vi "Connect Channel Command.vi"(8 "error in":errorcluster, 10 "Channel Connection Data":T1 {"Connection Data" format="%x"}, 11 "CIFCorePlugin in":refnum<class "CIFCorePlugin.lvclass">) -> (0 "error out":errorcluster, 3 "CIFCorePlugin out":refnum<class "CIFCorePlugin.lvclass">)   [LabVIEW 2021, in "CIFCorePlugin.lvclass"]
uses:
  CIFCorePlugin.lvclass
  CIFCorePlugin.lvclass/CIFCorePlugin.ctl
  Typedef/gRPC to Main Commands.ctl
  7fb4bced-bf7d-48d6-a5d3-7671888d20d0.vi
  Typedef/gRPC to Main Command Payload.ctl
  Common/Typedef/Channel Connection Data.ctl
  Common/CIFCoreCommon.lvlib
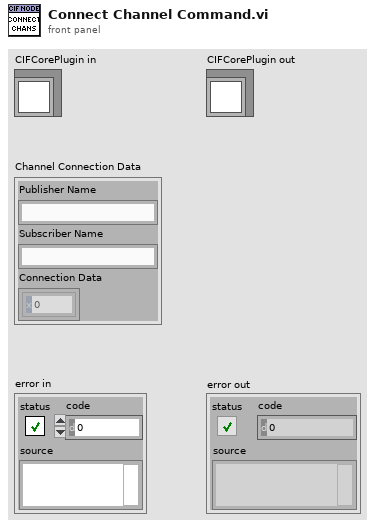
[diagram p1: front panel]
types:
  T1 = typedef "CIFCoreCommon.lvlib/Channel Connection Data.ctl" = cluster{"Publisher Name":string, "Subscriber Name":string, "Connection Data":u8[]}
  T2 = typedef "gRPC to Main Command Payload.ctl" = cluster{"OOB_Rx Command":T3, "Array Index":i32}
  T3 = typedef "CIFCorePlugin.lvclass/gRPC to Main Commands.ctl" = enum8{"Start", "Pause", "Stop", "RefreshStats", "UpdateConfig", "Update Clock Map", "Connect Channel", "Force Channel", "Add Publisher Instance", "Remove Publisher Instance"}
  T4 = typedef "CIFCorePlugin.lvclass/gRPC to Main DVR.ctl" = refnum<data-value>
  T5 = typedef "CIFCoreCommon.lvlib/gRPC to Main Data.ctl" = cluster{"Config Data":variant, "Connections":T1[], "Forces":T6[], "Clock Conversion":T7, "Publisher Instance":T9}
  T6 = typedef "CIFCoreCommon.lvlib/Channel Force Data.ctl" = cluster{"Channel Name":string, "Force Data":u8[], "Force Active":bool}
  T7 = typedef "Time_CIF_U.lvlib/Clock Conversion Map.ctl" = map{u8, cluster{"Last Reset":i64, "Offset Pair":T8, "Slope":dbl, "1/Slope":dbl}}
  T8 = typedef "Time_CIF_U.lvlib/Timestamp Pair.ctl" = cluster{"System Time":i64, "External Time":i64}
  T9 = typedef "CIFCoreCommon.lvlib/FIFO Publisher.ctl" = cluster{"Publisher Name":string, "New FIFO Instance Config":T10}
  T10 = typedef "ChannelCommon.lvlib/New FIFO Instance Configuration.ctl" = cluster{"Primary":bool, "Backpressure":bool, "Message/FIFO Override":u32}
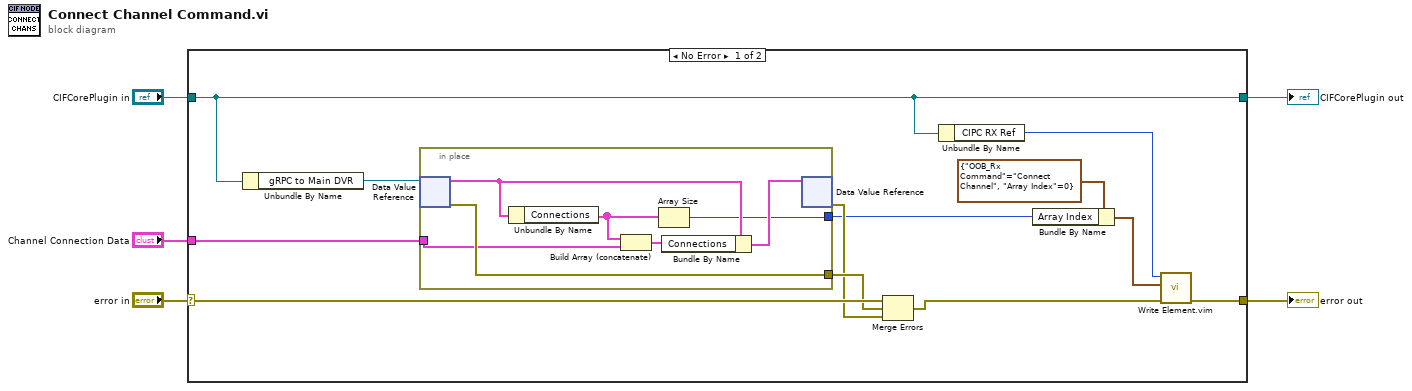
[diagram p0: block diagram]
diagram:
  n1 = case shown="No Error" "error in" {
    selector: "error in" -> [w12 w26]
    tunnel: [w17 w26] -> w4
    tunnel: "CIFCorePlugin in" -> [w15 w25]
    tunnel: [w15 w25] -> w2
    tunnel: "Channel Connection Data" -> [w13 _]
    frame No Error {
      n2 = Unbundle By Name(w15) -> ("gRPC to Main DVR"=w14:T4)
      n3 = in-place {
        in-place-border: w13 -> [w21]
        in-place-border: [w23] -> w11
        in-place-border: [w18] -> w7
        n4 = in-place-dvr #1(w14) -> (w22:T5, w23:errorcluster)
        n5 = Unbundle By Name(w22) -> ("Connections"=w19:T1[])
        n6 = Build Array (concatenate)(w19, w21) -> (w20:T1[])
        n7 = Array Size(array=w19) -> (size(s)=w18:i32)
        n8 = Bundle By Name(cluster=w22, "Connections"=w20) -> (w24:T5)
        n9 = in-place-dvr #1(w24) -> (w10:errorcluster)  [unwired: 1 out]
      }
      n10 = Merge Errors(w12, w11, w10) -> (w9:errorcluster)
      n11 = Unbundle By Name(w15) -> ("CIPC RX Ref"=w16:u64)
      n12 = Bundle By Name(cluster=T2 {"OOB_Rx Command"=enum."Connect Channel", "Array Index"=0} ("gRCP to Main Command Payload"), "Array Index"=w7) -> (w6:T2)
      n13 = call "Write Element.vim"("error in (no error)"=w9, "Data in"=w6, "CIPC Reference in"=w16) -> ("error out"=w17:errorcluster)  [unwired: 5 in, 3 out]
    }
    frame Error {
    }
  }
  "error out" <- w4
  "CIFCorePlugin out" <- w2
